vi "AH_GetSTB.vi"(8 "error in (no error)":errorcluster, 10 "Data Cluster In":T1 {"GUI Data Cluster"."SBR" format="%08b"}, 11 "Config Cluster In":T3={"General"={"Config.ini"=path "", "Default Logging Path"=path ""}, "Hardware"={"Measure Rate (1/s)"=0, "HP DMM VISA"="", "LS 335 VISA"="", "HP DM"={"Range"=enum."Autorange", "Autozero"=FALSE, "Display"=enum."3 1/2 Digit", "Blank LCD"=FALSE}}, "Operation"={"Operation Mode"=enum."Logging", "Status"="", "NewLog?"=FALSE, "OvenWarn"=FALSE}}) -> (0 "error out":errorcluster, 2 "Data Cluster Out":T1 {"GUI Data Cluster"."SBR" format="%08b"}, 3 "Configuration Cluster Out":T3={"General"={"Config.ini"=path "", "Default Logging Path"=path ""}, "Hardware"={"Measure Rate (1/s)"=0, "HP DMM VISA"="", "LS 335 VISA"="", "HP DM"={"Range"=enum."Autorange", "Autozero"=FALSE, "Display"=enum."3 1/2 Digit", "Blank LCD"=FALSE}}, "Operation"={"Operation Mode"=enum."Idle-Off", "Status"="", "NewLog?"=FALSE, "OvenWarn"=FALSE}})   [LabVIEW 2021]
uses:
  Mode_Enum.ctl
  Config_Cluster.ctl
  Measurement_Cluster.ctl
  Data_Cluster.ctl
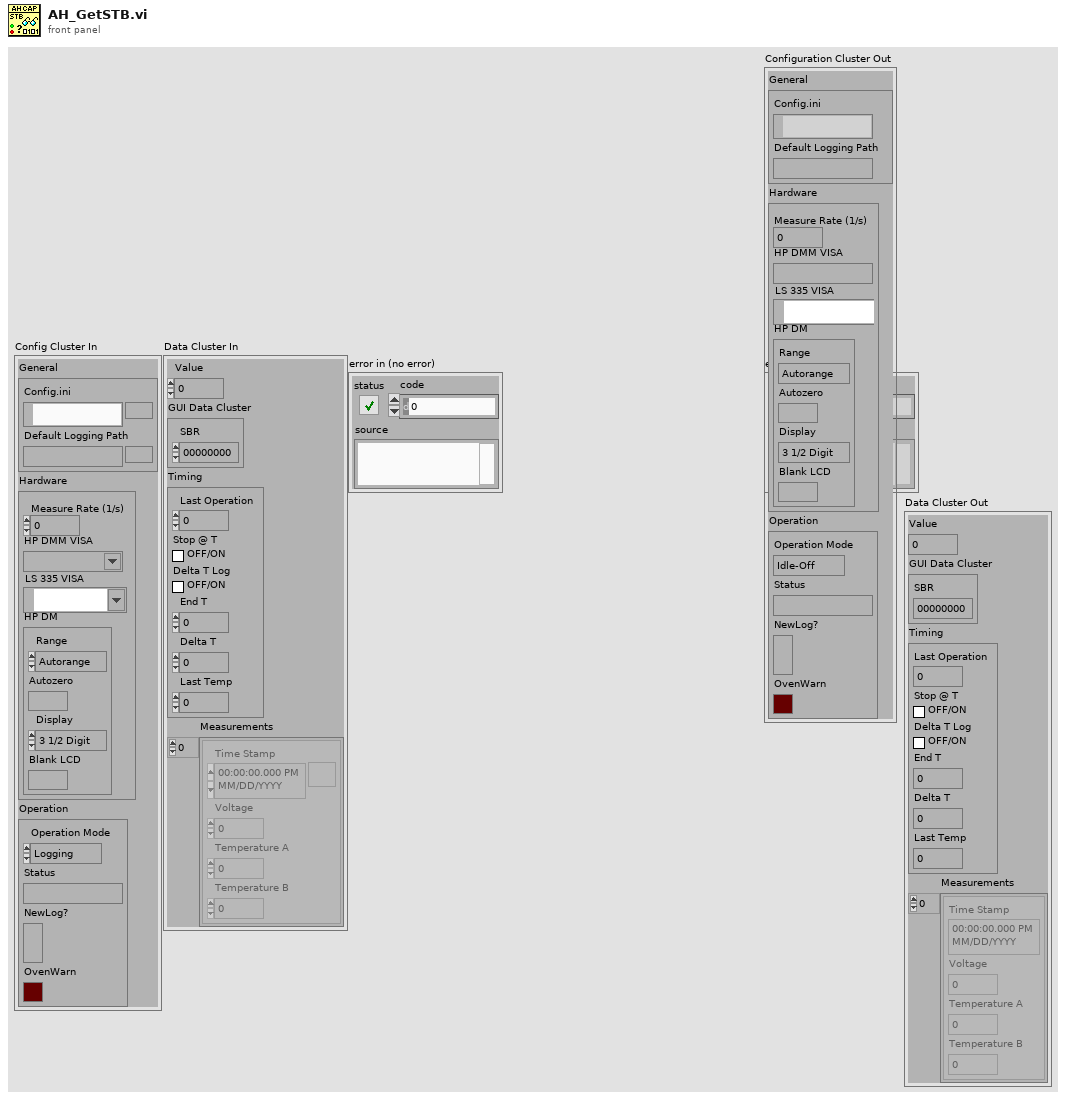
[diagram p1: front panel]
types:
  T1 = typedef "Data_Cluster.ctl" = cluster{"Value":dbl, "GUI Data Cluster":cluster{"SBR":u16}, "Timing":cluster{"Last Operation":dbl, "Stop @ T":bool, "Delta T Log":bool, "End T":dbl, "Delta T":dbl, "Last Temp":dbl}, "Measurements":T2[]}
  T2 = typedef "Measurement_Cluster.ctl" = cluster{"Time Stamp":timestamp, "Voltage":dbl, "Temperature A":dbl, "Temperature B":dbl}
  T3 = typedef "Config_Cluster.ctl" = cluster{"General":cluster{"Config.ini":path, "Default Logging Path":path}, "Hardware":cluster{"Measure Rate (1/s)":i32, "HP DMM VISA":refnum<visa-resource-name>, "LS 335 VISA":refnum<visa-resource-name>, "HP DM":cluster{"Range":enum16{"Autorange", "30mV", "300mV", "3V", "30V"}, "Autozero":bool, "Display":enum16{"3 1/2 Digit", "4 1/2 Digit", "5 1/2 Digit"}, "Blank LCD":bool}}, "Operation":cluster{"Operation Mode":T4, "Status":string, "NewLog?":bool, "OvenWarn":bool}}
  T4 = typedef "Mode_Enum.ctl" = enum16{"OvenNRDY", "Logging", "Idle-Off", "Idle"}
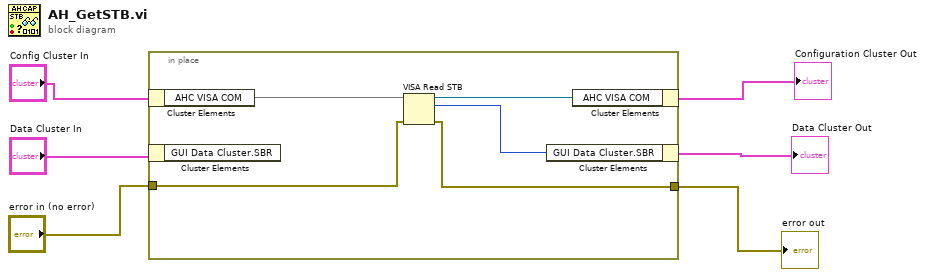
[diagram p0: block diagram]
diagram:
  n1 = in-place {
    in-place-border: "error in (no error)" -> [w8]
    in-place-border: [w7] -> w3
    n2 = in-place-cluster #1("Config Cluster In") -> ("AHC VISA COM"=w11)
    n3 = in-place-cluster #2("Data Cluster In") -> ()  [unwired: 1 out]
    n4 = VISA Read STB(8:w8, 11:w11) -> (0:w7:errorcluster, 2:w9:u16, 3:w10:refnum<visa-resource-name>)
    n5 = in-place-cluster #2("GUI Data Cluster.SBR"=w9) -> (→"Data Cluster Out":T1)
    n6 = in-place-cluster #1("AHC VISA COM"=w10) -> (→"Configuration Cluster Out":T3)
  }
  "error out" <- w3
